vi "Filters.vi"() -> ()   [LabVIEW 2016]
uses:
  controls/EnumFGVHDT.ctl
  controls/Enum.ctl
  <vilib>/addons/Digital Filter Design/_Objects.llb/DFD Filter Obj.ctl
  <vilib>/addons/Digital Filter Design/_Objects.llb/DFD Filter Coef.ctl
  <vilib>/addons/Digital Filter Design/_Objects.llb/DFD Filter Structure Type Selector.ctl
  <vilib>/addons/Digital Filter Design/_Objects.llb/dfd_Internal Quantization Settings.ctl
  <vilib>/addons/Digital Filter Design/_Objects.llb/dfd_Internal Quantization Srcs.ctl
  <vilib>/addons/Digital Filter Design/_Objects.llb/DFD Coef Norm Type.ctl
  <vilib>/addons/Digital Filter Design/_Objects.llb/DFD Plot Settings.ctl
  <vilib>/rvi/errors/niLvFpgaAdjustHostInterfaceError.vi
  <vilib>/addons/Digital Filter Design/Analysis.llb/DFD Plot Freq Response (Log-Spaced).vi
  <vilib>/regexp/Match Regular Expression.xnode
  <vilib>/rvi/interface/nirviReadWriteControl/nirviReadWriteControl.xnode
  controls/FPGAVIreferenceTypeDef.ctl
  FPGA Bitfiles/lbniAFMControlle_flexRio_controllerFPGA.lvbitx
  Course Project/support/Message Queue/Message Queue.lvlib
  <vilib>/addons/Digital Filter Design/NI_DigFilterLicensed.lvlib
  NiFpgaLv.dll
panel:
  in  "Activate ZFilter":bool=TRUE
  in  "Activate InputFilter":bool=TRUE
  in  "Sample Freq":dbl=1000000.0 min=0.001 format="%#_4pHz"
  in  "Z smoothing":T1={"Frequency"=100000.0, "Filter order"=2, "Type"=enum."Butterworth"} {"Frequency" min=0.001 max=500000000.0 format="%#_4p"}
  in  "InputFilter":T1={"Frequency"=100000.0, "Filter order"=2, "Type"=enum."Butterworth"} {"Frequency" min=0.001 max=500000000.0 format="%#_4p"}
  out "Reverse Coefficients 2":dbl[](array[numeric])
  out "Forward Coefficients 2":dbl[](array[numeric])
  out "Real":u32 format="%.0pHz"
  out "phase response":cluster{"bins":dbl[], "response FXP":dbl[]}[](graph)
  out "magnitude response":cluster{"bins":dbl[], "response FXP":dbl[]}[](graph)
  out "Forward Coefficients":dbl[](array[numeric])
  out "Reverse Coefficients":dbl[](array[numeric])
  in  "Output rate":dbl=500000.0 min=0.001 format="%#_4pS/s"
  # "Z smoothing"
  # "Input LP Filter AI0"
  # "(IO Rate)"
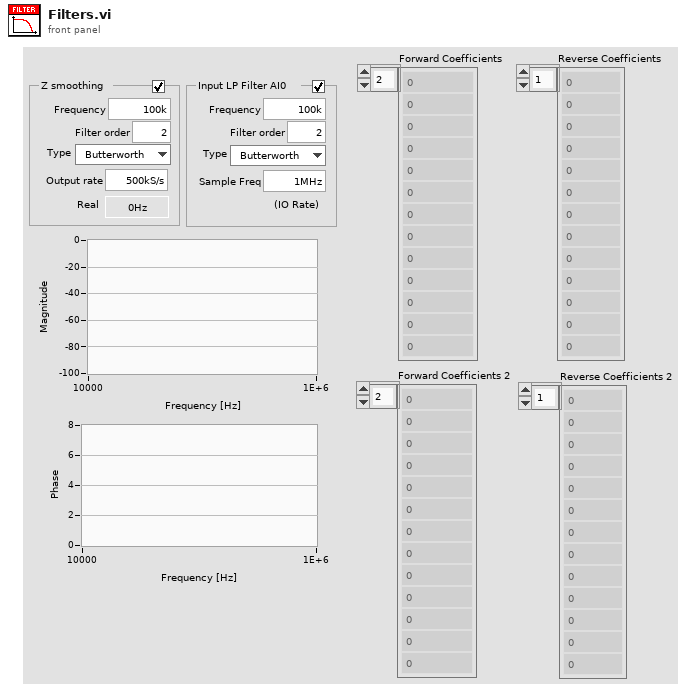
[diagram p1: front panel]
types:
  T1 = cluster{"Frequency":dbl, "Filter order":i32, "Type":enum16{"Butterworth", "Bessel"}}
  T2 = typedef "EnumFGVHDT.ctl" = enum16{"Init", "Read", "Write", "Push", "Pop"}
  T3 = typedef "Message Queue.lvlib/All Message Queues.ctl" = cluster{"IU":refnum<queue>}
  T4 = typedef "Enum.ctl" = enum16{"Init", "Read", "Write"}
  T5 = enum16{"Lowpass", "Highpass", "Bandpass", "Bandstop"}
  T6 = typedef "NI_DigFilterLicensed.lvlib/DFD Filter Obj.ctl" = cluster{"mSRate_Fs":dbl, "mSRate_Version":string, "mSRate_Comments":string, "mSRate_OrgCoef":T7, "mSRate_CurCoef":T7, "mSRate_Quantized?":bool, "mSRate_QCoef":T7, "mSRate_QSettings":T9[], "mSRate_Order":i32, "mSRate_Scaling":cluster{"mSRate_ScaleByPowerOf2?":bool, "mSRate_ScaleType":T11}}
  T7 = typedef "NI_DigFilterLicensed.lvlib/DFD Filter Coef.ctl" = cluster{"type":T8, "gain":dbl, "coef a (k)":dbl[], "coef b (v)":dbl[]}
  T8 = typedef "NI_DigFilterLicensed.lvlib/DFD Filter Structure Type Selector.ctl" = enum16{"Undefined", "FIR Direct Form", "FIR Direct Form Transposed", "FIR Symmetric", "FIR Antisymmetric", "IIR Direct Form I", "IIR Direct Form I Transposed", "IIR Direct Form II", "IIR Direct Form II Transposed", "IIR Cascaded Second Order Sections Form I", "IIR Cascaded Second Order Sections Form I Transposed", "IIR Cascaded Second Order Sections Form II", "IIR Cascaded Second Order Sections Form II Transposed", "Lattice Allpass (basic sections)", "Lattice Allpass (one multiplier sections)", "Lattice Allpass (normalized sections)", "Lattice AR (basic sections)", "Lattice AR (one multiplier sections)", "Lattice AR (normalized sections)", "Lattice MA (minimum phase)", "Lattice MA (maximum phase)", "Lattice ARMA (basic sections)", "Lattice ARMA (one multiplier sections)", "Lattice ARMA (normalized sections)"}
  T9 = typedef "NI_DigFilterLicensed.lvlib/dfd_Internal Quantization Settings.ctl" = cluster{"source":T10, "wl":i16, "iwl":i16, "overflow mode":enum16{"Saturation", "Wrap"}, "rounding mode":enum16{"Nearest", "Truncation"}, "signed?":bool}
  T10 = typedef "NI_DigFilterLicensed.lvlib/dfd_Internal Quantization Srcs.ctl" = u16
  T11 = typedef "NI_DigFilterLicensed.lvlib/DFD Coef Norm Type.ctl" = enum16{"No Norm", "Time Domain 1-Norm", "Time Domain 2-Norm", "Time Domain Inf-Norm"}
  T12 = typedef "NI_DigFilterLicensed.lvlib/DFD Plot Settings.ctl" = cluster{"# freq bins":i32, "low frequency [Hz]":dbl, "high frequency [Hz]":dbl}
  T13 = typedef "FPGAVIreferenceTypeDef.ctl" = refnum<k20>
  T14 = cluster{"filter structure":enum32{"IIR 2nd Order", "IIR 4th Order"}, "Reverse Coefficients":dbl[], "Forward Coefficients":dbl[]}
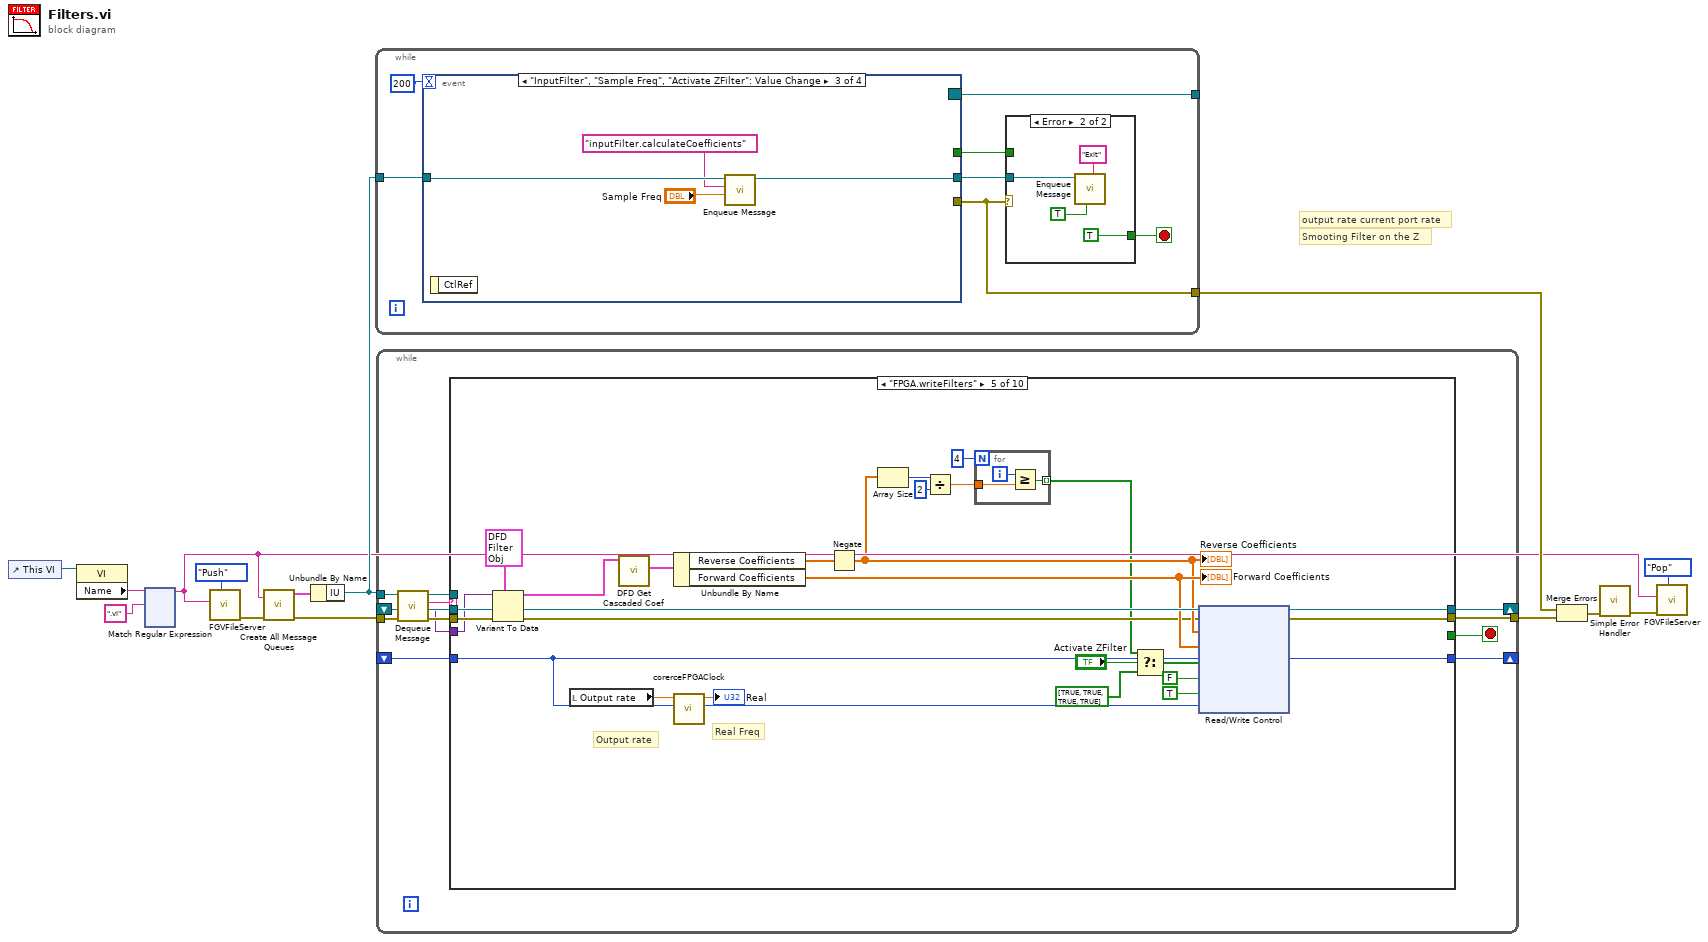
[diagram p0: block diagram]
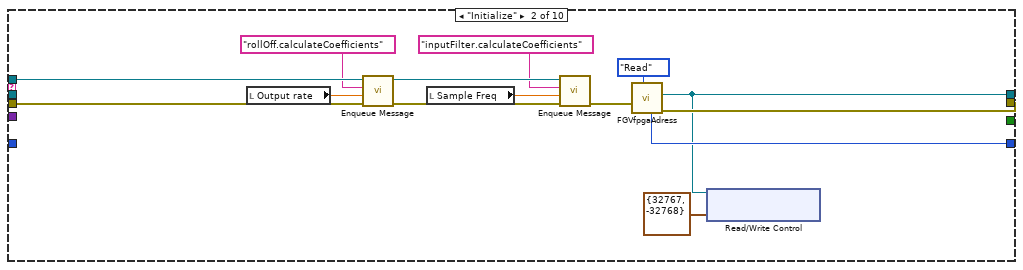
[diagram p3: hidden frame]
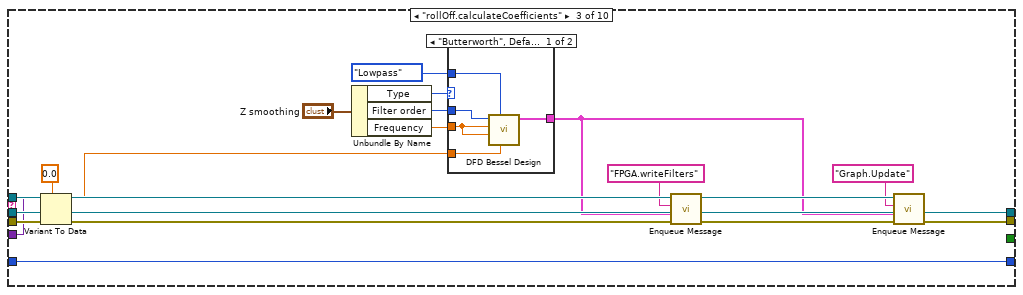
[diagram p4: hidden frame]
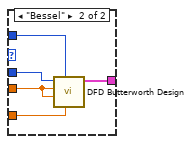
[diagram p5: hidden frame]
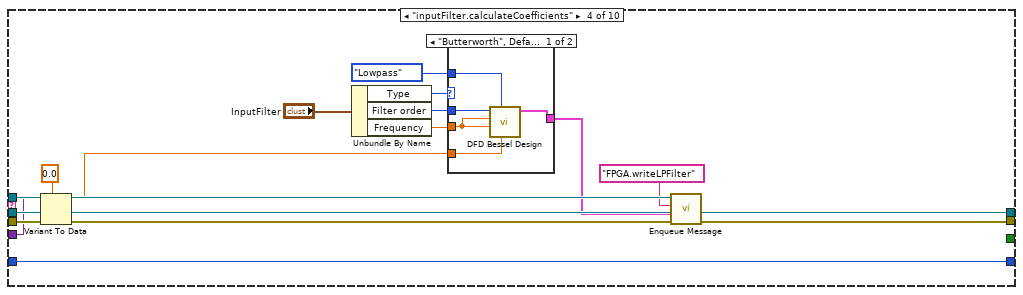
[diagram p6: hidden frame]
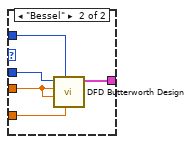
[diagram p7: hidden frame]
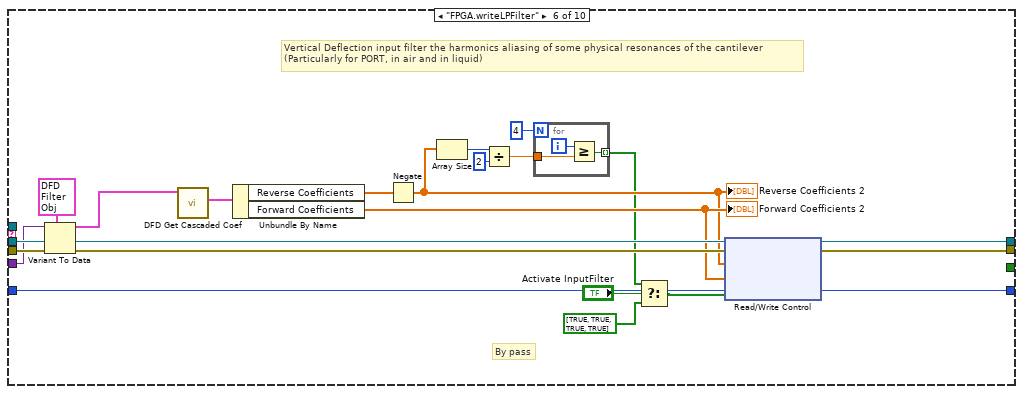
[diagram p8: hidden frame]
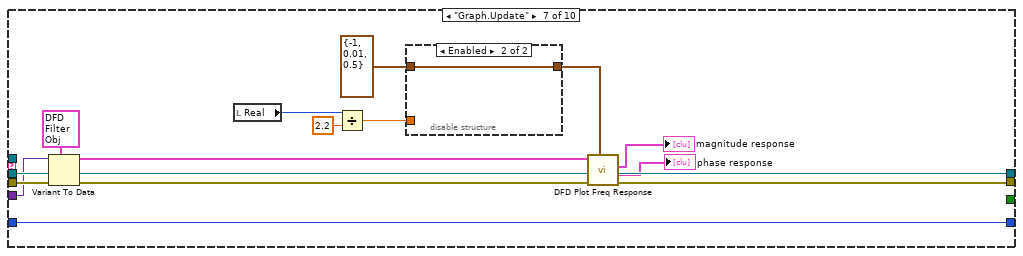
[diagram p9: hidden frame]
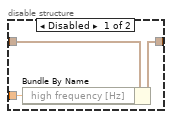
[diagram p10: hidden frame]
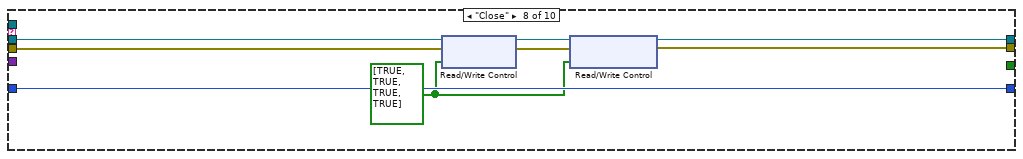
[diagram p11: hidden frame]
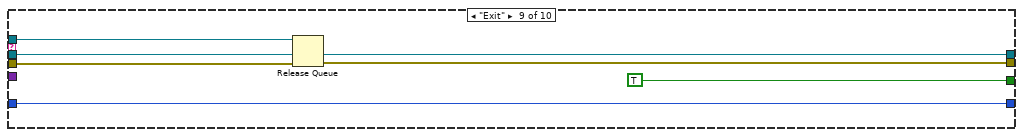
[diagram p12: hidden frame]
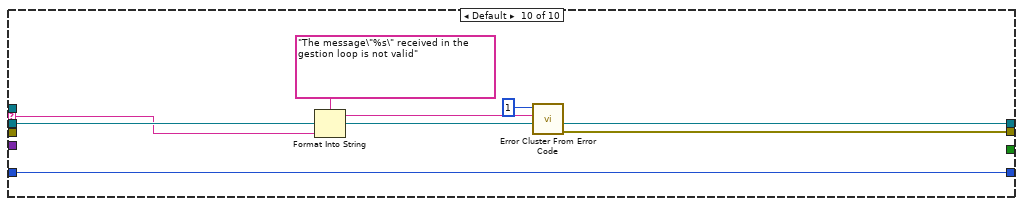
[diagram p13: hidden frame]
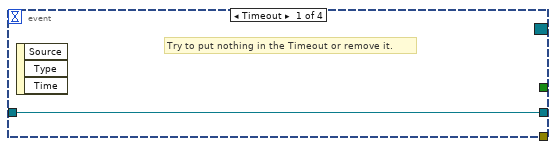
[diagram p15: hidden frame]
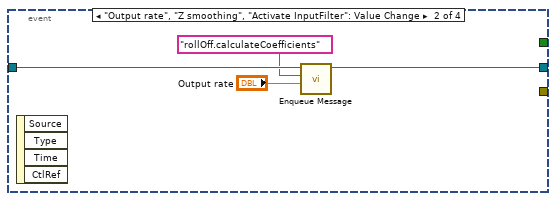
[diagram p16: hidden frame]
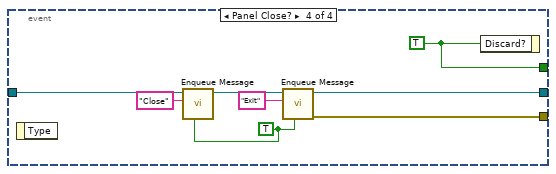
[diagram p17: hidden frame]
diagram:
  # "Smooting Filter on the Z"
  # "output rate current port rate"
  n1 = control-ref of="This VI"() -> (w4:refnum<vi>)
  n2 = property class="VI"(reference=w4) -> ("Name"=w3:string)  [unwired: 1 in, 2 out]
  n3 = xnode "Match Regular Expression"("input string"=w3, "regular expression"=".vi") -> ("before match"=w1:string)  [unwired: 4 in, 4 out]
  n4 = call "FGVFileServer.vi"("Enum"=EnumFGVHDT."Push", "New VI"=w1) -> ("error out"=w5:errorcluster)  [unwired: 8 in, 1 out]
  n5 = call "Create All Message Queues.vi"("QueueName"=w1, "ErrorIn"=w5) -> ("ErrorOut"=w12:errorcluster, "MessageQueueOut"=w14:T3)  [unwired: 8 in]
  n6 = Unbundle By Name(w14) -> ("IU"=w13:refnum<queue>)
  n7 = while {
    tunnel: w13 -> [w21]
    tunnel: [w17] -> w9
    tunnel: [w16] -> _
    stop <- w19 stop-if-true
    n8 = event shown="[2] \"InputFilter\", \"Sample Freq\", \"Activate ZFilter\": Value Change" {
      selector: _ -> [_ _ _ _]
      dyn-events: [_ _ _ _] -> w16
      timeout: 200 -> [_ _ _ _]
      tunnel: [_ _ _ w43] -> w20
      tunnel: w21 -> [w27 w31 w35 w39]
      tunnel: [_ _ _ w42] -> w17
      tunnel: [w27 w29 w33 w41] -> w18
      event Timeout {
        # "Try to put nothing in the Timeout or remove it."
        n9 = event-data() -> ()  [unwired: 1 in, 3 out]
      }
      event "Output rate", "Z smoothing", "Activate InputFilter": Value Change {
        n10 = event-data() -> ()  [unwired: 1 in, 4 out]
        n11 = call "Enqueue Message.vi"("Data"="Output rate", "Message"="rollOff.calculateCoefficients", "Queue"=w31) -> ("Queue dup."=w29:refnum<queue>)  [unwired: 7 in, 1 out]
      }
      event "InputFilter", "Sample Freq", "Activate ZFilter": Value Change {
        n12 = event-data() -> ()  [unwired: 1 in, 1 out]
        n13 = call "Enqueue Message.vi"("Data"="Sample Freq", "Message"="inputFilter.calculateCoefficients", "Queue"=w35) -> ("Queue dup."=w33:refnum<queue>)  [unwired: 7 in, 1 out]
      }
      event Panel Close? {
        w36 = TRUE ("Message prioritaire ? (F)")
        w43 = TRUE ("Rejeter ?")
        n14 = event-data() -> ()  [unwired: 1 in, 1 out]
        n15 = call "Enqueue Message.vi"("Prioritary message"=w36, "Message"="Close", "Queue"=w39) -> ("Queue dup."=w38:refnum<queue>)  [unwired: 7 in, 1 out]
        n16 = call "Enqueue Message.vi"("Prioritary message"=w36, "Message"="Exit", "Queue"=w38) -> ("error out"=w42:errorcluster, "Queue dup."=w41:refnum<queue>)  [unwired: 7 in]
        n17 = event-data ("Event Filter Node")("Discard?"=w43) -> ()  [unwired: 1 in, 1 out]
      }
    }
    n18 = case shown="Error" w17 {
      tunnel: [w22 TRUE ("Rejeter ?")] -> w19
      tunnel: w20 -> [w22 _]
      tunnel: w18 -> [_ w25]
      frame No Error {
      }
      frame Error {
        n19 = call "Enqueue Message.vi"("Prioritary message"=TRUE ("Message prioritaire ? (F)"), "Message"="Exit", "Queue"=w25) -> ()  [unwired: 7 in, 2 out]
      }
    }
  }
  n20 = while {
    tunnel: w13 -> [w50]
    tunnel: w12 -> [w53]
    tunnel: [w54] -> w10
    shift-right: [w47] -> _
    shift-left: _ -> [w48]
    shift-right: [w46] -> _
    shift-left: _ -> [w45]
    stop <- w55 stop-if-true
    n21 = call "Dequeue Message.vi"("entrée d'erreur (pas d'erreur)"=w53, "File d'attente de messages"=w50) -> ("sortie d'erreur"=w52:errorcluster, "Données de message"=w44:variant, "Message"=w49:string, "File d'attente de message dup."=w51:refnum<queue>)  [unwired: 6 in]
    n22 = case "Conditions des messages" shown="\"FPGA.writeFilters\"" w49 {
      selector: w49 -> [_ _ _ _ _ _ _ _ _ w218]
      tunnel: w51 -> [_ w71 w90 w117 _ _ _ _ w213 _]
      tunnel: w52 -> [w58 w68 w83 w112 w136 w163 w185 w203 w211 _]
      tunnel: [w58 w61 w86 w103 w148 w173 w181 w201 w210 w216] -> w54
      tunnel: [_ _ _ _ _ _ _ _ TRUE _] -> w55
      tunnel: w48 -> [w57 _ w88 w115 w149 w174 w195 w204 w209 w220]
      tunnel: [w57 w60 w88 w115 w147 w172 w195 w202 w209 w220] -> w47
      tunnel: [w56 w67 w87 w114 w144 w171 w194 w207 w208 w214] -> w46
      tunnel: w45 -> [w56 _ w87 w114 w144 w171 w194 w207 w208 w214]
      tunnel: w44 -> [_ _ w80 w109 w134 w161 w184 _ _ _]
      frame "--------- Initialization ---------" {
      }
      frame "Initialize" {
        n23 = local read "Output rate"() -> (w66:dbl)
        n24 = call "Enqueue Message.vi"("error in"=w68, "Data"=w66, "Message"="rollOff.calculateCoefficients", "Queue"=w71) -> ("error out"=w64:errorcluster, "Queue dup."=w72:refnum<queue>)  [unwired: 6 in]
        n25 = local read "Sample Freq"() -> (w62:dbl)
        n26 = call "Enqueue Message.vi"("error in"=w64, "Data"=w62, "Message"="inputFilter.calculateCoefficients", "Queue"=w72) -> ("error out"=w63:errorcluster)  [unwired: 6 in, 1 out]
        n27 = call "FGVfpgaAdress.vi"("Enum"=Enum."Read", "error in"=w63) -> ("error out"=w61:errorcluster, "FPGA VI Reference Out"=w60:T13, "ioFreqHzOut"=w67:u32)  [unwired: 4 in, 3 out]
        n28 = xnode "Read/Write Control"("FPGA VI Reference In"=w60, "aio.o.heightLimits"=cluster{"upper":i16, "lower":i16} {"upper"=32767, "lower"=-32768}) -> ()  [unwired: 1 in, 2 out]
      }
      frame "rollOff.calculateCoefficients" {
        n29 = Variant To Data(error in=w83, type=0.0 ("Output rate"), Variant=w80) -> (data=w79:dbl, error out=w82:errorcluster)
        n30 = Unbundle By Name("Z smoothing") -> ("Type"=w77:enum16{"Butterworth", "Bessel"}, "Filter order"=w76:i32, "Frequency"=w75:dbl)
        n31 = case shown="\"Butterworth\", Default" w77 {
          tunnel: w75 -> [w93 w97]
          tunnel: w76 -> [w95 w101]
          tunnel: T5."Lowpass" ("filter type") -> [w94 w100]
          tunnel: w79 -> [w92 w99]
          tunnel: [w96 w98] -> w73
          frame "Butterworth", Default {
            n32 = call <vilib>:"DFD Bessel Design.vi"("fs [Hz]"=w92, "filter type"=w94, "low cutoff freq [Hz]"=w93, "high cutoff freq [Hz]"=w93, "order"=w95) -> ("filter out"=w96:T6)  [unwired: 5 in, 1 out]
          }
          frame "Bessel" {
            n33 = call <vilib>:"DFD Butterworth Design.vi"("fs [Hz]"=w99, "filter type"=w100, "low cutoff freq [Hz]"=w97, "high cutoff freq [Hz]"=w97, "order"=w101) -> ("filter out"=w98:T6)  [unwired: 5 in, 1 out]
          }
        }
        n34 = call "Enqueue Message.vi"("error in"=w82, "Data"=w73, "Message"="FPGA.writeFilters", "Queue"=w90) -> ("error out"=w74:errorcluster, "Queue dup."=w91:refnum<queue>)  [unwired: 6 in]
        n35 = call "Enqueue Message.vi"("error in"=w74, "Data"=w73, "Message"="Graph.Update", "Queue"=w91) -> ("error out"=w86:errorcluster)  [unwired: 6 in, 1 out]
      }
      frame "inputFilter.calculateCoefficients" {
        n36 = Variant To Data(error in=w112, type=0.0 ("Output rate"), Variant=w109) -> (data=w108:dbl, error out=w111:errorcluster)
        n37 = Unbundle By Name("InputFilter") -> ("Type"=w107:enum16{"Butterworth", "Bessel"}, "Filter order"=w106:i32, "Frequency"=w105:dbl)
        n38 = case shown="\"Butterworth\", Default" w107 {
          tunnel: w105 -> [w119 w123]
          tunnel: w106 -> [w121 w127]
          tunnel: T5."Lowpass" ("filter type") -> [w120 w126]
          tunnel: w108 -> [w118 w125]
          tunnel: [w122 w124] -> w104
          frame "Butterworth", Default {
            n39 = call <vilib>:"DFD Bessel Design.vi"("fs [Hz]"=w118, "filter type"=w120, "low cutoff freq [Hz]"=w119, "high cutoff freq [Hz]"=w119, "order"=w121) -> ("filter out"=w122:T6)  [unwired: 5 in, 1 out]
          }
          frame "Bessel" {
            n40 = call <vilib>:"DFD Butterworth Design.vi"("fs [Hz]"=w125, "filter type"=w126, "low cutoff freq [Hz]"=w123, "high cutoff freq [Hz]"=w123, "order"=w127) -> ("filter out"=w124:T6)  [unwired: 5 in, 1 out]
          }
        }
        n41 = call "Enqueue Message.vi"("error in"=w111, "Data"=w104, "Message"="FPGA.writeLPFilter", "Queue"=w117) -> ("error out"=w103:errorcluster)  [unwired: 6 in, 1 out]
      }
      frame "FPGA.writeFilters" {
        # "Real Freq"
        # "Output rate"
        n42 = Variant To Data(error in=w136, type=T6 {"mSRate_Fs"=1.0, "mSRate_Version"="2.0", "mSRate_Comments"="", "mSRate_OrgCoef"={"type"=enum."Undefined", "gain"=1.0, "coef a (k)"=[], "coef b (v)"=[]}, "mSRate_CurCoef"={"type"=enum."Undefined", "gain"=1.0, "coef a (k)"=[], "coef b (v)"=[]}, "mSRate_Quantized?"=FALSE, "mSRate_QCoef"={"type"=enum."Undefined", "gain"=1.0, "coef a (k)"=[], "coef b (v)"=[]}, "mSRate_QSettings"=[], "mSRate_Order"=0, "mSRate_Scaling"={"mSRate_ScaleByPowerOf2?"=FALSE, "mSRate_ScaleType"=enum."No Norm"}} ("filter out"), Variant=w134) -> (data=w132:T6, error out=w135:errorcluster)
        n43 = local read "Output rate"() -> (w146:dbl)
        n44 = call <vilib>:"DFD Get Cascaded Coef.vi"("filter in"=w132) -> ("IIR Filter Cluster"=w153:T14)  [unwired: 7 in, 3 out]
        n45 = Unbundle By Name(w153) -> ("Reverse Coefficients"=w152:dbl[], "Forward Coefficients"=w142:dbl[])
        "Forward Coefficients" <- w142
        n46 = call "corerceFPGAClock.vi"("baseClock"=w144, "requestedFrequency"=w146) -> ("decimation"=w145:u16, "realFrequency"=→"Real":dbl)  [unwired: 7 in, 1 out]
        n47 = Negate(x=w152) -> (-x=w141:dbl[])
        "Reverse Coefficients" <- w141
        n48 = Array Size(array=w141) -> (size(s)=w140:i32)
        n49 = Divide(x=w140, y=2) -> (x/y=w137:dbl)
        n50 = for {
          N: 4 -> [_]
          tunnel: w137 -> [w155]
          tunnel: [w154] -> w129 mode=indexing
          i -> [w156]
          n51 = Greater Or Equal?(x=w156, y=w155) -> (x >= y?=w154:bool)
        }
        n52 = Select(t=w129, s="Activate ZFilter", f=bool[] [TRUE, TRUE, TRUE, TRUE] ("aio.flt.bypass")) -> (s? t:f=w128:bool[])
        n53 = xnode "Read/Write Control"("FPGA VI Reference In"=w149, "error in"=w135, "flt.p.anot4x"=w141, "flt.p.b4x"=w142, "flt.bypass2"=w128, "flt.bypassPI"=FALSE, "flt.ss.p.enable"=TRUE, "flt.ss.p.rate"=w145) -> ("FPGA VI Reference Out"=w147:T13, "error out"=w148:errorcluster)
      }
      frame "FPGA.writeLPFilter" {
        # "By pass"
        # "Vertical Deflection input filter the harmonics aliasing of some physical resonances of the cantilever\n(Particularly for PORT, in air and in liquid)"
        n54 = Variant To Data(error in=w163, type=T6 {"mSRate_Fs"=1.0, "mSRate_Version"="2.0", "mSRate_Comments"="", "mSRate_OrgCoef"={"type"=enum."Undefined", "gain"=1.0, "coef a (k)"=[], "coef b (v)"=[]}, "mSRate_CurCoef"={"type"=enum."Undefined", "gain"=1.0, "coef a (k)"=[], "coef b (v)"=[]}, "mSRate_Quantized?"=FALSE, "mSRate_QCoef"={"type"=enum."Undefined", "gain"=1.0, "coef a (k)"=[], "coef b (v)"=[]}, "mSRate_QSettings"=[], "mSRate_Order"=0, "mSRate_Scaling"={"mSRate_ScaleByPowerOf2?"=FALSE, "mSRate_ScaleType"=enum."No Norm"}} ("filter out"), Variant=w161) -> (data=w162:T6, error out=w177:errorcluster)
        n55 = call <vilib>:"DFD Get Cascaded Coef.vi"("filter in"=w162) -> ("IIR Filter Cluster"=w176:T14)  [unwired: 7 in, 3 out]
        n56 = Unbundle By Name(w176) -> ("Reverse Coefficients"=w175:dbl[], "Forward Coefficients"=w170:dbl[])
        "Forward Coefficients 2" <- w170
        n57 = Negate(x=w175) -> (-x=w169:dbl[])
        "Reverse Coefficients 2" <- w169
        n58 = Array Size(array=w169) -> (size(s)=w168:i32)
        n59 = Divide(x=w168, y=2) -> (x/y=w165:dbl)
        n60 = for {
          N: 4 -> [_]
          tunnel: w165 -> [w179]
          tunnel: [w178] -> w158 mode=indexing
          i -> [w180]
          n61 = Greater Or Equal?(x=w180, y=w179) -> (x >= y?=w178:bool)
        }
        n62 = Select(t=w158, s="Activate InputFilter", f=bool[] [TRUE, TRUE, TRUE, TRUE] ("aio.flt.bypass")) -> (s? t:f=w157:bool[])
        n63 = xnode "Read/Write Control"("FPGA VI Reference In"=w174, "error in"=w177, "aio.flt.p.anot4x"=w169, "aio.flt.p.b4x"=w170, "aio.flt.bypass"=w157) -> ("FPGA VI Reference Out"=w172:T13, "error out"=w173:errorcluster)
      }
      frame "Graph.Update" {
        n64 = Variant To Data(error in=w185, type=T6 {"mSRate_Fs"=1.0, "mSRate_Version"="2.0", "mSRate_Comments"="", "mSRate_OrgCoef"={"type"=enum."Undefined", "gain"=1.0, "coef a (k)"=[], "coef b (v)"=[]}, "mSRate_CurCoef"={"type"=enum."Undefined", "gain"=1.0, "coef a (k)"=[], "coef b (v)"=[]}, "mSRate_Quantized?"=FALSE, "mSRate_QCoef"={"type"=enum."Undefined", "gain"=1.0, "coef a (k)"=[], "coef b (v)"=[]}, "mSRate_QSettings"=[], "mSRate_Order"=0, "mSRate_Scaling"={"mSRate_ScaleByPowerOf2?"=FALSE, "mSRate_ScaleType"=enum."No Norm"}} ("filter out"), Variant=w184) -> (data=w183:T6, error out=w182:errorcluster)
        n65 = local read "Real"() -> (w189:u32)
        n66 = Divide(x=w189, y=2.2) -> (x/y=w187:dbl)
        n67 = disable-structure shown="Enabled" {
          disable-tunnel: T12 {"# freq bins"=-1, "low frequency [Hz]"=0.01, "high frequency [Hz]"=0.5} ("plot settings") -> [w198 w199]
          disable-tunnel: [w197 w199] -> w190
          disable-tunnel: w187 -> [w196 _]
          frame Disabled {
            n68 = Bundle By Name(cluster=w198, "high frequency [Hz]"=w196) -> (w197:T12)
          }
          frame Enabled {
          }
        }
        n69 = call-poly <vilib>:"DFD Plot Freq Response.vi"("plot settings"=w190, "error in (no error)"=w182, "filter in"=w183) -> ("error out"=w181:errorcluster, "phase response"=→"phase response":cluster{"bins":dbl[], "response FXP":dbl[]}[], "magnitude response"=→"magnitude response":cluster{"bins":dbl[], "response FXP":dbl[]}[])  [unwired: 5 in, 1 out]
      }
      frame "Close" {
        w200 = bool[] [TRUE, TRUE, TRUE, TRUE] ("aio.flt.bypass")
        n70 = xnode "Read/Write Control"("FPGA VI Reference In"=w204, "error in"=w203, "flt.bypass2"=w200) -> ("FPGA VI Reference Out"=w206:T13, "error out"=w205:errorcluster)
        n71 = xnode "Read/Write Control"("FPGA VI Reference In"=w206, "error in"=w205, "aio.flt.bypass"=w200) -> ("FPGA VI Reference Out"=w202:T13, "error out"=w201:errorcluster)
      }
      frame "Exit" {
        n72 = Release Queue(queue=w213, error in (no error)=w211) -> (error out=w210:errorcluster)  [unwired: 1 in, 2 out]
      }
      frame Default {
        n73 = Format Into String(format string="The message\"%s\" received in the gestion loop is not valid" ("Texte de message d'erreur inconnu"), w218) -> (resulting string=w215:string)  [unwired: 2 in, 1 out]
        n74 = call <vilib>:"Error Cluster From Error Code.vi"("error message (\"\")"=w215, "error code (0)"=1 ("code d'erreur (0)")) -> ("error out"=w216:errorcluster)  [unwired: 7 in]
      }
    }
  }
  n75 = Merge Errors(w9, w10) -> (w11:errorcluster)
  n76 = call <vilib>:"Simple Error Handler.vi"("error in (no error)"=w11) -> ("error out"=w7:errorcluster)  [unwired: 4 in, 4 out]
  n77 = call "FGVFileServer.vi"("Enum"=EnumFGVHDT."Pop", "error in"=w7, "New VI"=w1) -> ()  [unwired: 7 in, 2 out]
